vi "DAQ.Clear.vi"(8 "error in (no error)":errorcluster, 11 "Instrument.DAQ in":refnum<class "Instrument.DAQ.lvclass">) -> (0 "error out":errorcluster, 3 "Instrument.DAQ out":refnum<class "Instrument.DAQ.lvclass">)   [LabVIEW 2019, in "Instrument.Lockin.lvlib" / "Instrument.DAQ.lvclass"]
uses:
  Instrument.DAQ.lvclass
  Instrument.DAQ.lvclass/Instrument.DAQ.ctl
  DAQmx/DAQmx.lvclass
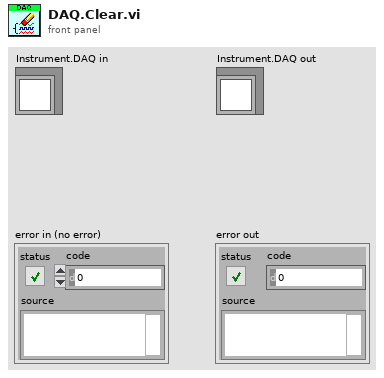
[diagram p1: front panel]
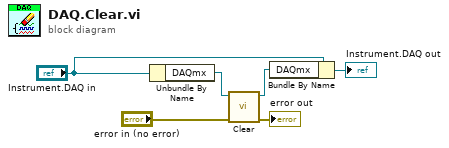
[diagram p0: block diagram]
diagram:
  n1 = Unbundle By Name("Instrument.DAQ in") -> ("DAQmx"=w4:refnum<class "DAQmx.lvclass">)
  n2 = call "Clear.vi"("error in (no error)"="error in (no error)", "DAQmx in"=w4) -> ("error out"=→"error out":errorcluster, "DAQmx out"=w3:refnum<class "DAQmx.lvclass">)  [unwired: 8 in]
  n3 = Bundle By Name(cluster="Instrument.DAQ in", "DAQmx"=w3) -> (→"Instrument.DAQ out":refnum<class "Instrument.DAQ.lvclass">)
